vi "Trilinear - Supporting Function.vi"(9 "Z":dbl, 10 "Y":dbl, 11 "X":dbl) -> (3 "C Array":dbl[](array[numeric]))   [LabVIEW 2019]
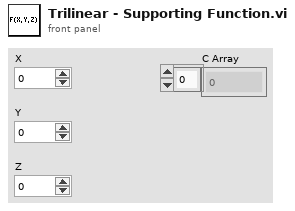
[diagram p1: front panel]
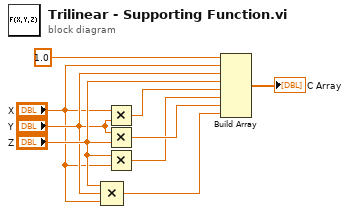
[diagram p0: block diagram]
diagram:
  n1 = Compound Arithmetic op=MULTIPLY("Z", "Y", "X") -> (w7:dbl)
  n2 = Multiply(x="X", y="Y") -> (x*y=w3:dbl)
  n3 = Multiply(x="Y", y="Z") -> (x*y=w9:dbl)
  n4 = Multiply(x="Z", y="X") -> (x*y=w8:dbl)
  n5 = Build Array(1.0 ("element"), "X", "Y", "Z", w3, w8, w9, w7) -> (→"C Array":dbl[])
